vi "Generate Service Request.vi"(4 "error in (no error)":errorcluster, 6 "Interrupt Number (0)":i32 min=0 max=31, 7 "VISA resource name":refnum<visa-resource-name>) -> (0 "error out":errorcluster, 3 "VISA resource name out":refnum<visa-resource-name>)   [LabVIEW 2018, in "Newport ESP301.lvlib"]
doc: "This command generates an interrupt service request to the host computer. The parameter Interrupt Number (0) is used to identify the RQ command which generated the interrupt. Upon receiving the interrupt, the host computer interrupt service routine should perform an IEEE 488 serial poll. If the interrupt was as a result of the RQ command, then bit 6 of the response is 1 and the lower five bits equal the parameter Interrupt Number (0).\nThis command can be used to notify the host computer of the progress or flow of command execution in the motion controller."
uses:
  Newport ESP301.lvlib
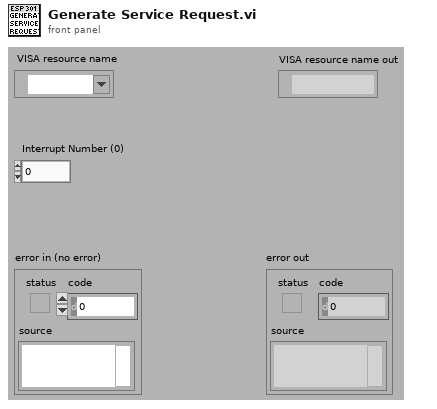
[diagram p1: front panel]
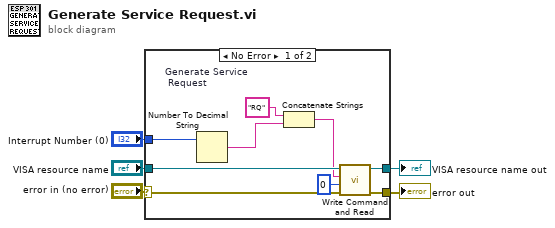
[diagram p0: block diagram]
diagram:
  n1 = case shown="No Error" "error in (no error)" {
    selector: "error in (no error)" -> [w11 w16]
    tunnel: [w13 w16] -> w5
    tunnel: "VISA resource name" -> [w14 w15]
    tunnel: [w12 w15] -> w4
    tunnel: "Interrupt Number (0)" -> [w8 _]
    frame No Error {
      w10 = "RQ"  # Generate Service  Request
      n2 = Number To Decimal String(number=w8) -> (decimal integer string=w6:string)  [unwired: 1 in]
      n3 = Concatenate Strings(w10, w6) -> (w9:string)
      n4 = call "Write Command and Read.vi"("error in (no error)"=w11, "Bytes to read (100)"=u32 0, "Command"=w9, "VISA resource name"=w14) -> ("error out"=w13:errorcluster, "VISA resource name out"=w12:refnum<visa-resource-name>)  [unwired: 3 in, 1 out]
    }
    frame Error {
    }
  }
  "error out" <- w5
  "VISA resource name out" <- w4
